vi "variant1.vi"() -> ()   [LabVIEW 2016]
panel:
  out "values 2":bool
  out "values":string
  out "data":dbl
  in  "variant":variant
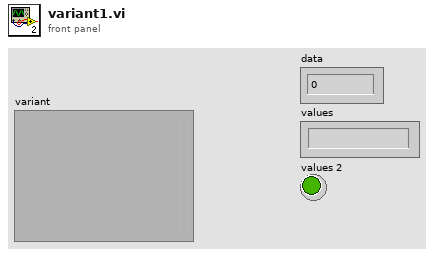
[diagram p1: front panel]
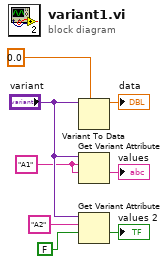
[diagram p0: block diagram]
diagram:
  w4 = "A1" ("name")
  n1 = Variant To Data(type=0.0, Variant="variant") -> (data=→"data":dbl)  [unwired: 1 in, 1 out]
  n2 = Get Variant Attribute(Variant="variant", name=w4, default value (empty Variant)=w4) -> (value=→"values":string)  [unwired: 1 in, 3 out]
  n3 = Get Variant Attribute(Variant="variant", name="A2", default value (empty Variant)=FALSE) -> (value=→"values 2":bool)  [unwired: 1 in, 3 out]
